vi "Fdx Start (Rx).vi"(8 "error in":errorcluster, 11 "InstrumentHandle_port in":u32) -> (0 "error out":errorcluster, 3 "InstrumentHandle_port out":u32)   [LabVIEW 2020, in "AIM664LV.lvlib"]
doc: "This function is used to start the receive operation of the board."
uses:
  AIM664LV.lvlib
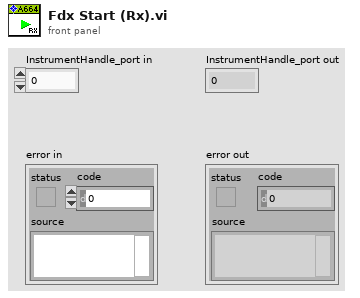
[diagram p1: front panel]
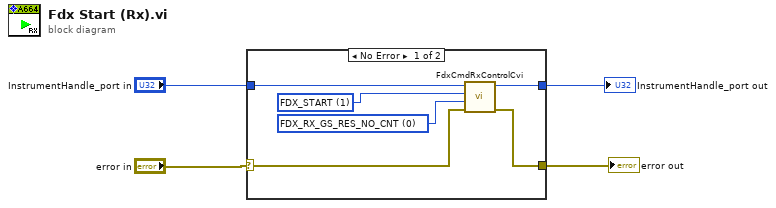
[diagram p0: block diagram]
diagram:
  n1 = case shown="No Error" "error in" {
    selector: "error in" -> [w10 w11]
    tunnel: "InstrumentHandle_port in" -> [w8 w12]
    tunnel: [w9 w11] -> w2
    tunnel: [w5 w12] -> w1
    frame No Error {
      w7 = u32 1 items=["FDX_STOP", "FDX_START"] ("StartMode")
      w6 = u32 0 items=["FDX_RX_GS_RES_NO_CNT", "FDX_RX_GS_RES_ALL_CNT", "FDX_RX_GS_RES_ERR_CNT "] ("GlobalStatisticReset")
      n2 = call "FdxCmdRxControlCvi.vi"("error in"=w10, "GlobalStatisticReset"=w6, "StartMode"=w7, "InstrumentHandle_port in"=w8) -> ("error out"=w9:errorcluster, "InstrumentHandle_port out"=w5:u32)  [unwired: 6 in]
    }
    frame Error {
    }
  }
  "error out" <- w2
  "InstrumentHandle_port out" <- w1
